vi "SaveFPObjectConfiguration.vi"(0 "FP Name":string, 2 "Objects Configurations":T1[](array[typedef]), 5 "error in (no error)":errorcluster) -> (19 "error out":errorcluster)   [LabVIEW 2014, in "FrontPanelPublisher.lvlib" / "WebFrontPanel.lvclass"]
uses:
  WebFrontPanel.lvclass
  Controls/FPObjectConfiguration.ctl
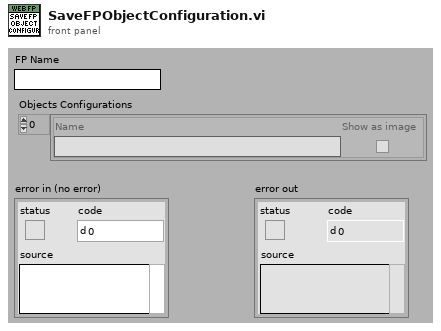
[diagram p1: front panel]
types:
  T1 = typedef "FrontPanelPublisher.lvlib/WebFrontPanel.lvclass/FPObjectConfiguration.ctl" = cluster{"Name":string, "Show as image":bool}
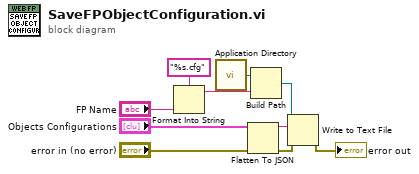
[diagram p0: block diagram]
diagram:
  n1 = Format Into String(format string="%s.cfg", "FP Name") -> (resulting string=w7:string)  [unwired: 2 in, 1 out]
  n2 = call <vilib>:"Application Directory.vi"() -> ("Application Directory"=w9:path)
  n3 = Flatten To JSON(anything="Objects Configurations", error in (no error)="error in (no error)") -> (JSON string=w2:string, 11:w3:errorcluster)  [unwired: 1 in]
  n4 = Build Path(base path=w9, name or relative path=w7) -> (appended path=w5:path)
  n5 = Write to Text File(file (use dialog)=w5, text=w2, error in=w3) -> (error out=→"error out":errorcluster)  [unwired: 1 in, 2 out]
